vi "new_DMM.vi"() -> ()   [LabVIEW 2009]
panel:
  out "Waveform Chart":dynamicdata(graph)
  out "output 1":dbl
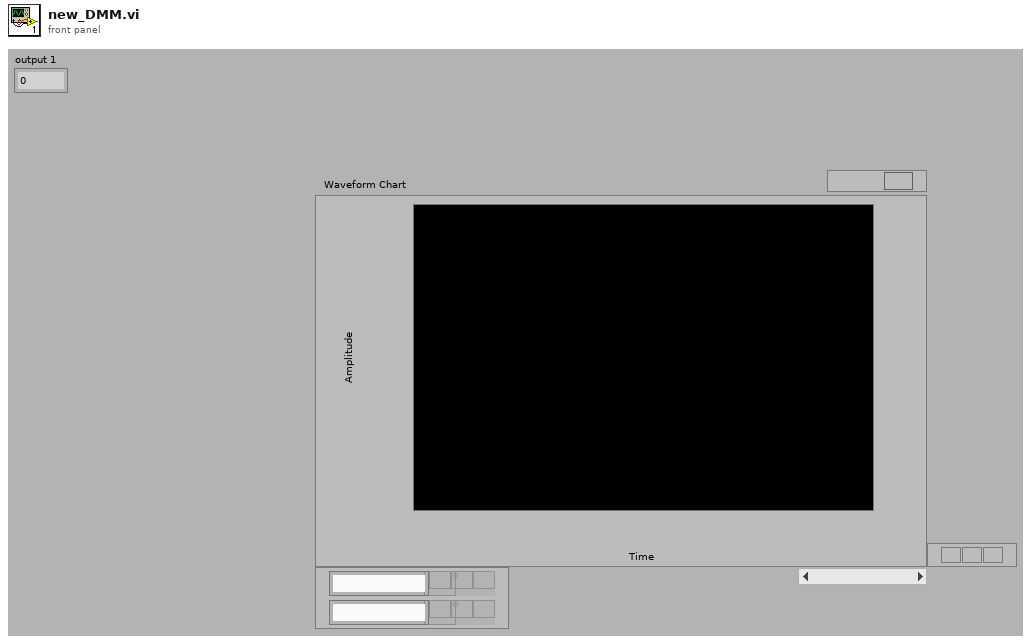
[diagram p1: front panel]
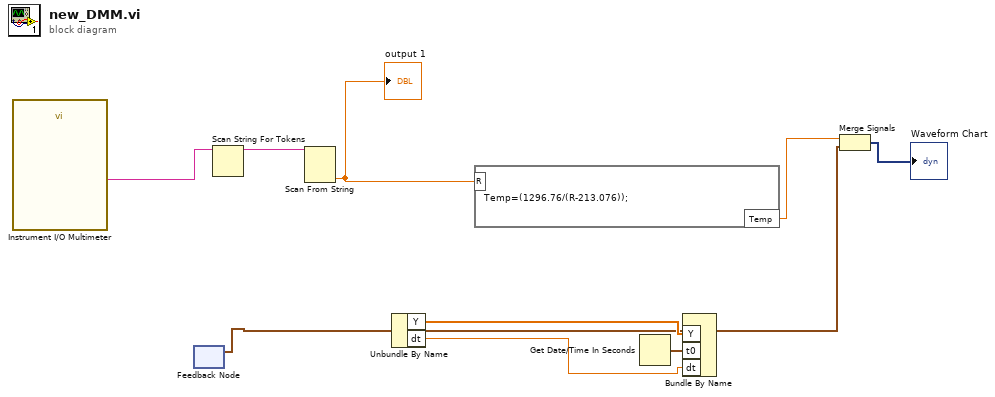
[diagram p0: block diagram]
diagram:
  n1 = call "Instrument I/O Multimeter"() -> ("Sample rate"=w10:string)  [unwired: 25 in, 2 out]
  n2 = feedback #1() -> (w2:waveform(dbl))  [unwired: 1 in]
  n3 = Scan String For Tokens(9:w10) -> (3:w9:string)  [unwired: 5 in, 3 out]
  n4 = Scan From String(input string=w9) -> (output 1=w8:dbl)  [unwired: 4 in, 3 out]
  "output 1" <- w8
  n5 = Unbundle By Name(w2) -> ("Y"=w6:dbl[], "dt"=w7:dbl)
  n6 = formula code="Temp=(1296.76/(R-213.076));"("R"=w8) -> ("Temp"=w3:dbl)
  n7 = Get Date/Time In Seconds() -> (seconds since 1Jan1904=w5:timestamp)
  n8 = Bundle By Name("Y"=w6, "t0"=w5, "dt"=w7) -> (w4:waveform(dbl))  [unwired: 1 in]
  n9 = Merge Signals(w3, w2) -> (→"Waveform Chart":dynamicdata)
